vi "Strip INI File.vi"(8 "error in (no error)":errorcluster, 10 "create file if necessary? (F)":bool, 11 "appended path":path) -> (0 "error out":errorcluster, 1 "Data":cluster{"Keys":string[], "Values":string[]}[](array[cluster]), 2 "section names":string[](array[string]))   [LabVIEW 2017]
uses:
  <vilib>/Utility/config.llb/Read Key (String).vi
  <vilib>/Utility/config.llb/NI_LVConfig.lvlib
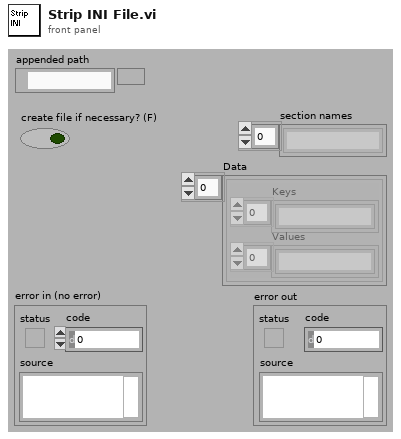
[diagram p1: front panel]
types:
  T1 = typedef "NI_LVConfig.lvlib/Config Data RefNum.ctl" = refnum<k1>
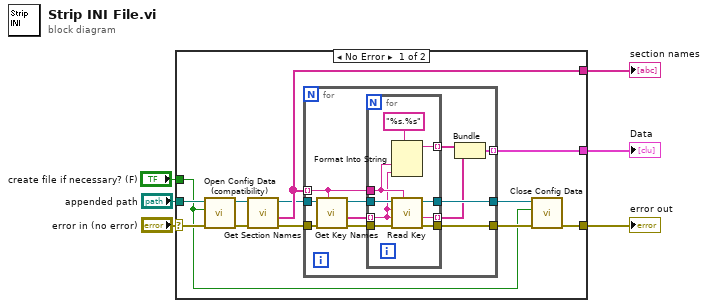
[diagram p0: block diagram]
diagram:
  n1 = case shown="No Error" "error in (no error)" {
    selector: "error in (no error)" -> [w8 w39]
    tunnel: "appended path" -> [w18 _]
    tunnel: [w17 _] -> w5
    tunnel: [w16 _] -> w4
    tunnel: [w15 w39] -> w3
    tunnel: "create file if necessary? (F)" -> [w7 _]
    frame No Error {
      n2 = call <vilib>:"Open Config Data (compatibility).vi"("error in (no error)"=w8, "create file if necessary (T)"=w7, "configuration file path"=w18) -> ("error out"=w14:errorcluster, "refnum"=w13:T1)  [unwired: 6 in, 1 out]
      n3 = call <vilib>:"Get Section Names.vi"("error in (no error)"=w14, "refnum"=w13) -> ("error out"=w12:errorcluster, "section names"=w17:string[], "refnum out"=w11:T1)  [unwired: 7 in]
      n4 = for {
        tunnel: w12 -> [w29]
        tunnel: w11 -> [w28]
        tunnel: w17 -> [w25] mode=indexing
        tunnel: [w24] -> w10
        tunnel: [w23] -> w9
        tunnel: [w19] -> w16 mode=indexing
        n5 = call <vilib>:"Get Key Names.vi"("section"=w25, "error in (no error)"=w29, "refnum"=w28) -> ("error out"=w26:errorcluster, "key names"=w22:string[], "refnum out"=w27:T1)  [unwired: 5 in, 1 out]
        n6 = for {
          tunnel: w27 -> [w38]
          tunnel: w22 -> [w31] mode=indexing
          tunnel: [w37] -> w20 mode=indexing
          tunnel: [w36] -> w24
          tunnel: w26 -> [w35]
          tunnel: [w34] -> w23
          tunnel: w25 -> [w32]
          tunnel: [w30] -> w21 mode=indexing
          n7 = Format Into String(format string="%s.%s", w32, w31) -> (resulting string=w30:string)  [unwired: 2 in, 1 out]
          n8 = call-poly <vilib>:"Read Key.vi"("section"=w32, "error in (no error)"=w35, "default value"=w31, "key"=w31, "refnum"=w38) -> ("error out"=w34:errorcluster, "value"=w37:string, "refnum out"=w36:T1)  [unwired: 3 in, 1 out]
        }
        n9 = Bundle(w21, w20) -> (w19:cluster{string[], string[]})  [unwired: 1 in]
      }
      n10 = call <vilib>:"Close Config Data.vi"("error in (no error)"=w9, "write file if changed (T)"=w7, "refnum"=w10) -> ("error out"=w15:errorcluster)  [unwired: 7 in, 1 out]
    }
    frame Error {
    }
  }
  "section names" <- w5
  "Data" <- w4
  "error out" <- w3
